vi "test_generic.vi"() -> ()   [LabVIEW 2010, in "GenericClock.lvclass"]
uses:
  GenericClock.lvclass
  common/classes/GenericComponent/GenericComponent/GenericComponent.lvclass
panel:
  in  "Triggered?":bool
  out "source out":string
  out "message":string=" INSTRUCTIONS:\r\rNormal Use:  When using subVIs that incorporate the error in/error out (or error I/O) structure, place this handler where you want to inform the user of an error, typically at the end of the I/O data path, as the last action of the program.  If the error in error? is ERROR, the handler creates a message describing the error and its source.  If the type of dialog = 1 (default), the message is displayed to the user, who can only acknowedge it.  If the type = 2, the user can acknowledge the message or abort execution; aborting a program with active I/O is not recommended.  If the type = 0, no message is displayed; this is used to process the error programmatically, and the error out cluster elements are wired to individual terminals for that reason.  \r\rOther Use:\n\r\nlocal testing.  To test the error code of a subVI or function that does not have the error I/O structure, you can wire its error code and a source string to the local error code and error source inputs.  If error in error? indicates no error and error code is not equal to 0, the local code and source are substituted for the error in values, and error? is set TRUE (ERROR)."
  in  "repetition period":dbl[unit]=5.0
  in  "number of pulses":i32=100
  in  "offset":dbl[unit]=1.0
  in  "create button":bool
  out "error out":errorcluster
  in  "stop":bool
  in  "start":bool
  in  "number of repetitions":i64=100
  in  "pulse frequency":dbl[unit]=100.0
  # "Test GenericClock"
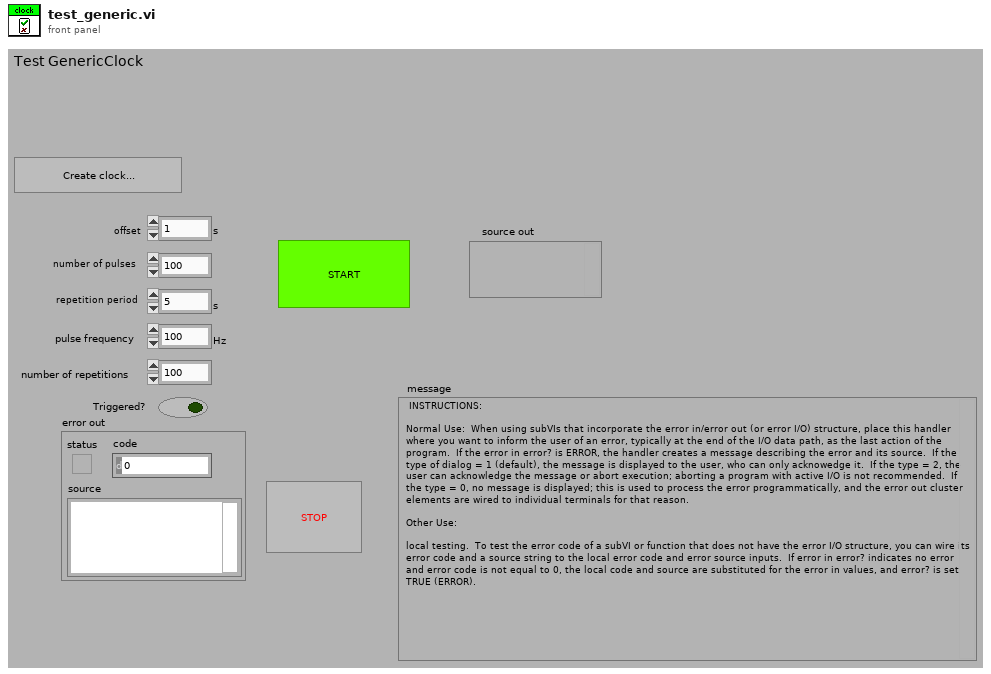
[diagram p1: front panel]
types:
  T1 = typedef "XComponentSpecification.xctl/data.ctl" = cluster{"class path":string, "configuration":string, "label":string, "settings name":string}
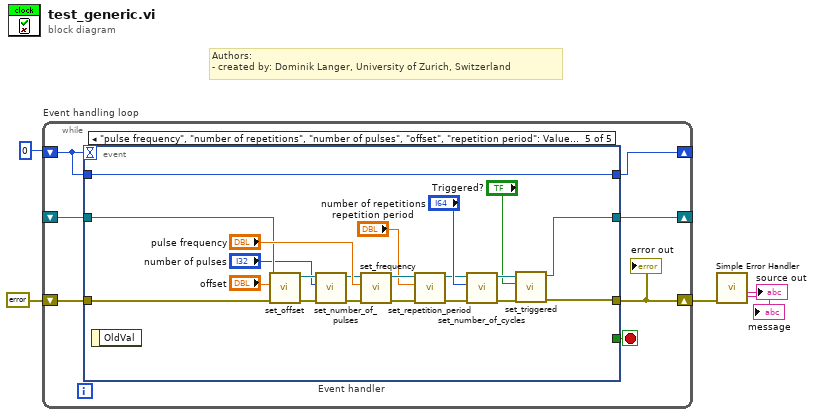
[diagram p0: block diagram]
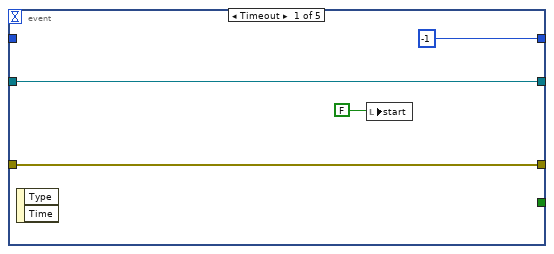
[diagram p2: hidden frame]
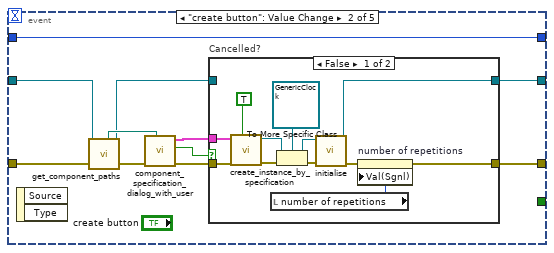
[diagram p3: hidden frame]
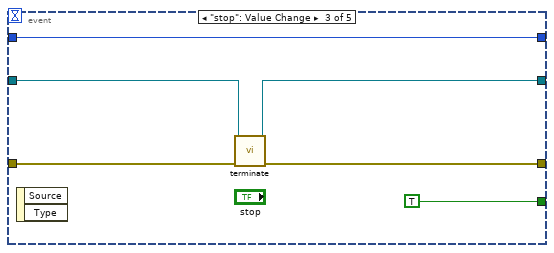
[diagram p5: hidden frame]
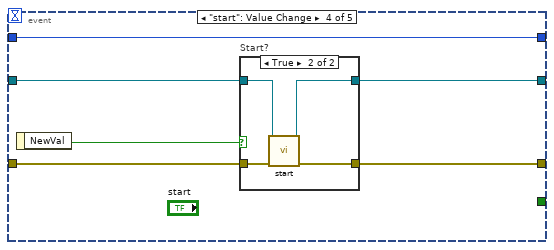
[diagram p6: hidden frame]
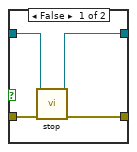
[diagram p7: hidden frame]
diagram:
  # "Authors: \n- created by: Dominik Langer, University of Zurich, Switzerland"
  n1 = while "Event handling loop" {
    shift-right: [w9] -> w3
    shift-left: errorcluster {"status"=FALSE, "code"=0, "source"=""} ("error out") -> [w10]
    shift-right: [w8] -> _
    shift-left: _ -> [w12]
    shift-right: [w7] -> _
    shift-left: 0 -> [w11]
    stop <- w6 stop-if-true
    n2 = event "Event handler" shown="[4] \"pulse frequency\", \"number of repetitions\", \"number of pulses\", \"offset\", \"repetition period\": Value Change" {
      selector: _ -> [_ _ _ _ _]
      dyn-events: _ -> [_ _ _ _ _]
      timeout: w11 -> [_ _ _ _ _]
      tunnel: w12 -> [w14 w21 w45 w51 w75]
      tunnel: w11 -> [_ w27 w47 w48 w80]
      tunnel: w10 -> [w13 w20 w44 w53 w78]
      tunnel: [w13 w26 w43 w50 w63] -> w9
      tunnel: [w14 w25 w42 w49 w64] -> w8
      tunnel: [-1 w27 w47 w48 w80] -> w7
      tunnel: [_ _ TRUE _ _] -> w6
      event Timeout {
        n3 = event-data() -> ()  [unwired: 3 out]
        n4 = local write "start"(FALSE) -> ()
      }
      event "create button": Value Change {
        n5 = event-data() -> ()  [unwired: 3 out]
        n6 = call-dynamic "get_component_paths.vi"("error in (no error)"=w20, "GenericComponent in"=w21) -> ("error out"=w19:errorcluster, "GenericComponent out"=w17:refnum<class "GenericClock.lvclass">, "component type directory"=w18:path)  [unwired: 4 in, 3 out]
        n7 = call "component_specification_dialog_with_user.vi"("start path"=w18, "error in (no error)"=w19) -> ("error out"=w24:errorcluster, "cancelled?"=w22:bool, "component specification out"=w23:T1)  [unwired: 7 in]
        n8 = case "Cancelled?" shown="False" w22 {
          tunnel: [w37 w40] -> w26
          tunnel: [w35 w41] -> w25
          tunnel: w24 -> [w29 w40]
          tunnel: w23 -> [w28 _]
          tunnel: w17 -> [_ w41]
          frame False {
            n9 = call "create_instance_by_specification.vi"("call constructor?"=TRUE, "error in (no error)"=w29, "component specification"=w28) -> ("error out"=w32:errorcluster, "GenericPlugin out"=w31:refnum<class "GenericComponent.lvclass">)  [unwired: 6 in, 1 out]
            n10 = local read "number of repetitions"() -> (w38:i64)
            n11 = To More Specific Class(target class=refnum<class "GenericClock.lvclass"> refnum ("GenericClock.lvclass"), reference=w31, error in=w32) -> (specific class reference=w33:refnum<class "GenericClock.lvclass">, error out=w34:errorcluster)
            n12 = call-dynamic "initialise.vi"("error in (no error)"=w34, "GenericPlugin in"=w33) -> ("error out"=w36:errorcluster, "GenericPlugin out"=w35:refnum<class "GenericClock.lvclass">)  [unwired: 8 out]
            n13 = property on="number of repetitions" class="DigNum (strict)"(error in=w36, "Val(Sgnl)"=w38) -> (error out=w37:errorcluster)  [unwired: 1 in, 1 out]
          }
          frame True {
          }
        }
      }
      event "stop": Value Change {
        n14 = event-data() -> ()  [unwired: 3 out]
        n15 = call-dynamic "terminate.vi"("error in (no error)"=w44, "GenericPlugin in"=w45) -> ("error out"=w43:errorcluster, "GenericPlugin out"=w42:refnum<class "GenericClock.lvclass">)  [unwired: 8 in]
      }
      event "start": Value Change {
        n16 = event-data() -> ("NewVal"=w52:bool)  [unwired: 1 out]
        n17 = case "Start?" shown="True" w52 {
          tunnel: w53 -> [w57 w61]
          tunnel: w51 -> [w56 w60]
          tunnel: [w54 w59] -> w50
          tunnel: [w55 w58] -> w49
          frame False {
            n18 = call-dynamic "stop.vi"("error in (no error)"=w57, "GenericClock in"=w56) -> ("error out"=w54:errorcluster, "GenericClock out"=w55:refnum<class "GenericClock.lvclass">)  [unwired: 8 out]
          }
          frame True {
            n19 = call-dynamic "start.vi"("error in (no error)"=w61, "GenericClock in"=w60) -> ("error out"=w59:errorcluster, "GenericClock out"=w58:refnum<class "GenericClock.lvclass">)  [unwired: 8 out]
          }
        }
      }
      event "pulse frequency", "number of repetitions", "number of pulses", "offset", "repetition period": Value Change {
        n20 = event-data() -> ()  [unwired: 2 out]
        n21 = call-dynamic "set_offset.vi"("error in (no error)"=w78, "offset"="offset", "GenericClock.lvclass in"=w75) -> ("error out"=w77:errorcluster, "GenericClock.lvclass out"=w76:refnum<class "GenericClock.lvclass">)  [unwired: 7 out]
        n22 = call-dynamic "set_number_of_pulses.vi"("error in (no error)"=w77, "number of pulses"="number of pulses", "GenericClock.lvclass in"=w76) -> ("error out"=w79:errorcluster, "GenericClock.lvclass out"=w74:refnum<class "GenericClock.lvclass">)  [unwired: 7 out]
        n23 = call-dynamic "set_frequency.vi"("error in (no error)"=w79, "frequency"="pulse frequency", "GenericClock.lvclass in"=w74) -> ("error out"=w69:errorcluster, "GenericClock.lvclass out"=w71:refnum<class "GenericClock.lvclass">)  [unwired: 7 out]
        n24 = call-dynamic "set_repetition_period.vi"("error in (no error)"=w69, "repetition period"="repetition period", "GenericClock.lvclass in"=w71) -> ("error out"=w68:errorcluster, "GenericClock.lvclass out"=w70:refnum<class "GenericClock.lvclass">)  [unwired: 7 out]
        n25 = call-dynamic "set_number_of_cycles.vi"("error in (no error)"=w68, "number of cycles"="number of repetitions", "GenericClock.lvclass in"=w70) -> ("error out"=w66:errorcluster, "GenericClock.lvclass out"=w65:refnum<class "GenericClock.lvclass">)  [unwired: 7 out]
        n26 = call-dynamic "set_triggered.vi"("error in (no error)"=w66, "triggered?"="Triggered?", "GenericClock.lvclass in"=w65) -> ("error out"=w63:errorcluster, "GenericClock.lvclass out"=w64:refnum<class "GenericClock.lvclass">)  [unwired: 7 in]
      }
    }
    "error out" <- w9
  }
  n27 = call <vilib>:"Simple Error Handler.vi"("error in (no error)"=w3) -> ("source out"=→"source out":string, "message"=→"message":string)  [unwired: 4 in, 3 out]
